vi "Reports.Results Chicony CSV Data to JSON Files.vi"(8 "error in (no error)":errorcluster, 9 "CSV Data File":path, 11 "Output Folder":path) -> (0 "error out":errorcluster)   [LabVIEW 2018]
uses:
  <vilib>/KATE/Files/File Utils.lvlib
panel:
  out "Record Cnt":i32
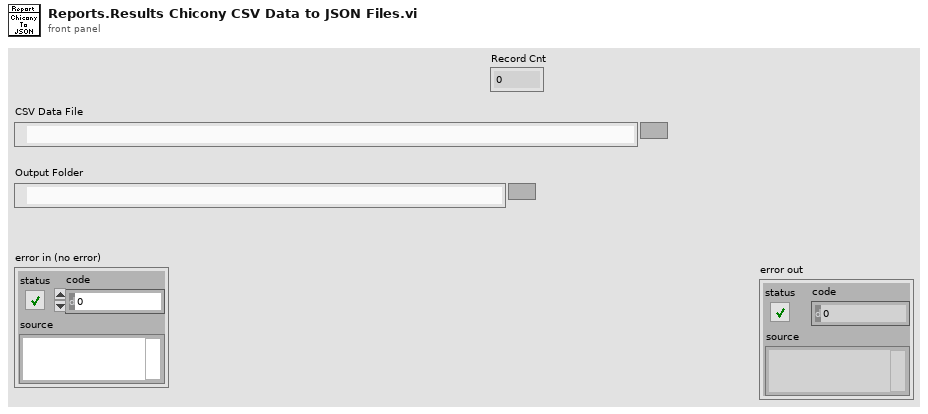
[diagram p1: front panel]
types:
  T1 = typedef "Report.Result Data JSON V2.0.0.ctl" = cluster{"Type":string, "Version":string, "TestEvent":T2, "UUTInfo":T4, "Station":T5, "TestSequence":T6, "NumericData":T7[], "AttributeData":T8[], "DataObjs":T9[]}
  T2 = typedef "Report.Result Test Event.ctl" = cluster{"ProcessStep":string, "StartTime":string, "EndTime":string, "Mode":string, "Operator":string, "Comment":string, "Result":T3}
  T3 = typedef "Report.Result State.ctl" = cluster{"State":string, "Code":i32, "Desc":string, "Details":string}
  T4 = typedef "Report.Result UUTInfo.ctl" = cluster{"PN":string, "SN":string, "LotNumber":string, "DateCode":string, "AltID":string, "Properties":cluster{"Name":string, "Value":string}[], "Revision":string}
  T5 = typedef "Report.Result Test Station.ctl" = cluster{"Name":string, "Location":string, "ConfigID":string, "PCName":string, "Slot":string}
  T6 = typedef "Report.Result Test Sequence.ctl" = cluster{"Name":string, "Setup":cluster{"Name":string, "Value":string}[]}
  T7 = typedef "Report.Result Numeric.ctl" = cluster{"Cnt":i32, "Step":string, "Category":string, "Name":string, "Value":dbl, "Units":string, "LimType":string, "LL":dbl, "UL":dbl, "Time":string, "Result":T3}
  T8 = typedef "Report.Result Attribute.ctl" = cluster{"Cnt":i32, "Step":string, "Category":string, "Name":string, "Value":string, "Units":string, "LimType":string, "LL":string, "UL":string, "Time":string, "Result":T3}
  T9 = typedef "Report.Result DataObject.ctl" = cluster{"Cnt":i32, "Step":string, "Category":string, "Name":string, "Type":string, "File Name":string, "Time":string}
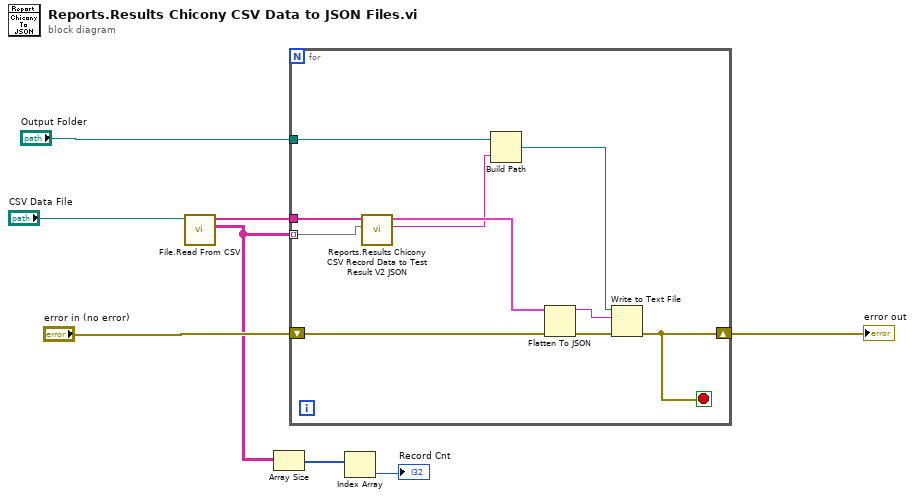
[diagram p0: block diagram]
diagram:
  n1 = call <vilib>:"File.Read From CSV.vi"("File"="CSV Data File") -> ("Data"=w3:string[][], "Header"=w5:string[])  [unwired: 8 in, 1 out]
  n2 = Array Size(array=w3) -> (size(s)=w2:i32[])
  n3 = for {
    tunnel: w5 -> [w12]
    shift-right: [w11] -> w7
    shift-left: "error in (no error)" -> [w16]
    tunnel: w3 -> [w10] mode=indexing
    tunnel: "Output Folder" -> [w9]
    stop <- w11 stop-if-true
    n4 = call "Reports.Results Chicony CSV Record Data to Test Result V2 JSON.vi"("Data"=w10, "Header"=w12) -> ("File Name"=w14:string, "Test Result V2.0.0"=w15:T1)  [unwired: 8 in]
    n5 = Build Path(base path=w9, name or relative path=w14) -> (appended path=w13:path)
    n6 = Flatten To JSON(anything=w15, error in (no error)=w16) -> (JSON string=w18:string, 11:w17:errorcluster)  [unwired: 1 in]
    n7 = Write to Text File(file (use dialog)=w13, text=w18, error in=w17) -> (error out=w11:errorcluster)  [unwired: 1 in, 2 out]
  }
  "error out" <- w7
  n8 = Index Array(array=w2) -> (element=→"Record Cnt":i32)  [unwired: 1 in]
